vi "Example.vi"   [LabVIEW 2026]
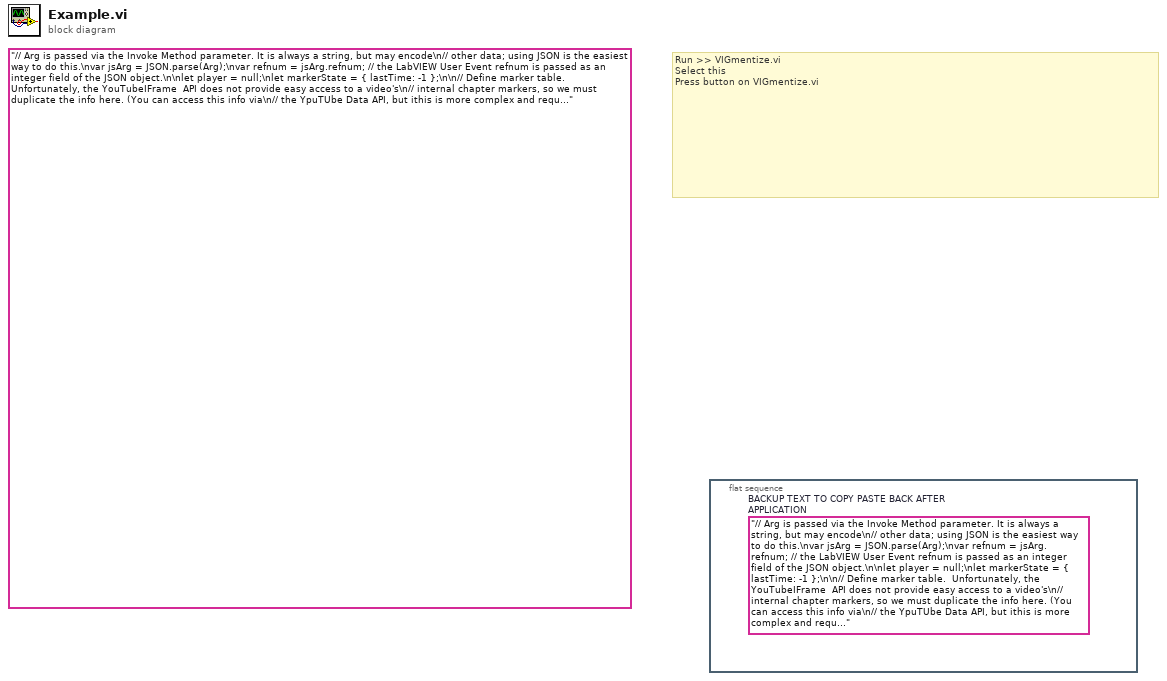
[diagram p0: block diagram]
diagram:
  (unwired) "// Arg is passed via the Invoke Method parameter. It is always a string, but may encode\n// other data; using JSON is the easiest way to do this.\nvar jsArg = JSON.parse(Arg);\nvar refnum = jsArg.refnum; // the LabVIEW User Event refnum is passed as an integer field of the JSON object.\n\nlet player = null;\nlet markerState = { lastTime: -1 };\n\n// Define marker table.  Unfortunately, the YouTubeIFrame  API does not provide easy access to a video's\n// internal chapter markers, so we must duplicate the info here. (You can access this info via\n// the YpuTUbe Data API, but ithis is more complex and requires an API key.)\nconst markers = [\n    { time: 0,   message: \"Playing Introduction\" },\n    { time: 13,  message: \"LabVIEW Interface\" },\n    { time: 34, message: \"Controls palette\" },\n    { time: 112,  message: \"String palette\" },\n    { time: 149,  message: \"String constant\" },\n    { time: 161,  message: \"Hello world!\" },\n    { time: 174,  message: \"Run\" },\n];\n\n// Pass a message to LabVIEW via a User event\nfunction notify(message) {\n    // The event will be handled by another case of the Event structure.\n    LabVIEW.FireUserEvent(refnum, message);\n}\n\n// Called when the YouTube player has finished initializing\nfunction onPlayerReady(event) {\n    // Stash the player in the global window object, so the 'Stop' event can stop the video;\n    // (ExecuteJavascript code executes in an anonymous function scope, so variables are\n    // not visible in other instances, but you can add them to existing global JS objects such\n    // as window in order to persist them between instances.)\n    window.player = player; \n\n    setInterval(() => {\n        if (!player || player.getPlayerState() !== YT.PlayerState.PLAYING)\n            return;\n\n        const now = player.getCurrentTime();\n        const last = markerState.lastTime;\n\n        // Check for crossed markers\n        for (const m of markers) {\n            if (last < m.time && now >= m.time) {\n                notify(m.message);\n            }\n        }\n        markerState.lastTime = now;\n    }, 100); // Polling interval (100ms)\n}\n\n// If this code was in the original referring web page, this function would be called automatically\n// by the IFrame API. \nfunction onYouTubeIframeAPIReady() {\n    player = new YT.Player('player', {\n        width: 640,\n        height: 360,\n        videoId: \"ZHNlKyYzrPE\",\n        playerVars: { // mute is needed because YT prevents programmatic autoplay of non-muted videos\n            rel: 0, autoplay : 1, mute: 1, playsinline: 1\n        },\n        events: {\n            'onReady': onPlayerReady\n        }\n    });\n}\n// Running this code in the Web Browser control's 'Load Finished' method also ensures\n// the API is ready, so we call the function directly.\nonYouTubeIframeAPIReady();\nreturn 0;\n" ("Javascript String")
  # "Run >> VIGmentize.vi\nSelect this\nPress button on VIGmentize.vi"
  n1 = flat-sequence {
    frame #0 {
      (unwired) "// Arg is passed via the Invoke Method parameter. It is always a string, but may encode\n// other data; using JSON is the easiest way to do this.\nvar jsArg = JSON.parse(Arg);\nvar refnum = jsArg.refnum; // the LabVIEW User Event refnum is passed as an integer field of the JSON object.\n\nlet player = null;\nlet markerState = { lastTime: -1 };\n\n// Define marker table.  Unfortunately, the YouTubeIFrame  API does not provide easy access to a video's\n// internal chapter markers, so we must duplicate the info here. (You can access this info via\n// the YpuTUbe Data API, but ithis is more complex and requires an API key.)\nconst markers = [\n    { time: 0,   message: \"Playing Introduction\" },\n    { time: 13,  message: \"LabVIEW Interface\" },\n    { time: 34, message: \"Controls palette\" },\n    { time: 112,  message: \"String palette\" },\n    { time: 149,  message: \"String constant\" },\n    { time: 161,  message: \"Hello world!\" },\n    { time: 174,  message: \"Run\" },\n];\n\n// Pass a message to LabVIEW via a User event\nfunction notify(message) {\n    // The event will be handled by another case of the Event structure.\n    LabVIEW.FireUserEvent(refnum, message);\n}\n\n// Called when the YouTube player has finished initializing\nfunction onPlayerReady(event) {\n    // Stash the player in the global window object, so the 'Stop' event can stop the video;\n    // (ExecuteJavascript code executes in an anonymous function scope, so variables are\n    // not visible in other instances, but you can add them to existing global JS objects such\n    // as window in order to persist them between instances.)\n    window.player = player; \n\n    setInterval(() => {\n        if (!player || player.getPlayerState() !== YT.PlayerState.PLAYING)\n            return;\n\n        const now = player.getCurrentTime();\n        const last = markerState.lastTime;\n\n        // Check for crossed markers\n        for (const m of markers) {\n            if (last < m.time && now >= m.time) {\n                notify(m.message);\n            }\n        }\n        markerState.lastTime = now;\n    }, 100); // Polling interval (100ms)\n}\n\n// If this code was in the original referring web page, this function would be called automatically\n// by the IFrame API. \nfunction onYouTubeIframeAPIReady() {\n    player = new YT.Player('player', {\n        width: 640,\n        height: 360,\n        videoId: \"ZHNlKyYzrPE\",\n        playerVars: { // mute is needed because YT prevents programmatic autoplay of non-muted videos\n            rel: 0, autoplay : 1, mute: 1, playsinline: 1\n        },\n        events: {\n            'onReady': onPlayerReady\n        }\n    });\n}\n// Running this code in the Web Browser control's 'Load Finished' method also ensures\n// the API is ready, so we call the function directly.\nonYouTubeIframeAPIReady();\nreturn 0;\n"  # BACKUP TEXT TO COPY PASTE BACK AFTER APPLICATION
    }
  }
